vi "lisa_functional_3.vi"   [LabVIEW 2019]
doc: "The classic \"Hello World\" example."
uses:
  <vilib>/Analysis/Matrix/Datatypes/ComplexMatrix.ctl
  <vilib>/Analysis/Matrix/NI_Matrix.lvlib
types:
  T1 = typedef "imagedata.ctl" = cluster{"image type":i32, "image depth":i32, "image":u8[], "mask":u8[], "colors":u32[], "Rectangle":cluster{"left":i16, "top":i16, "right":i16, "bottom":i16}}
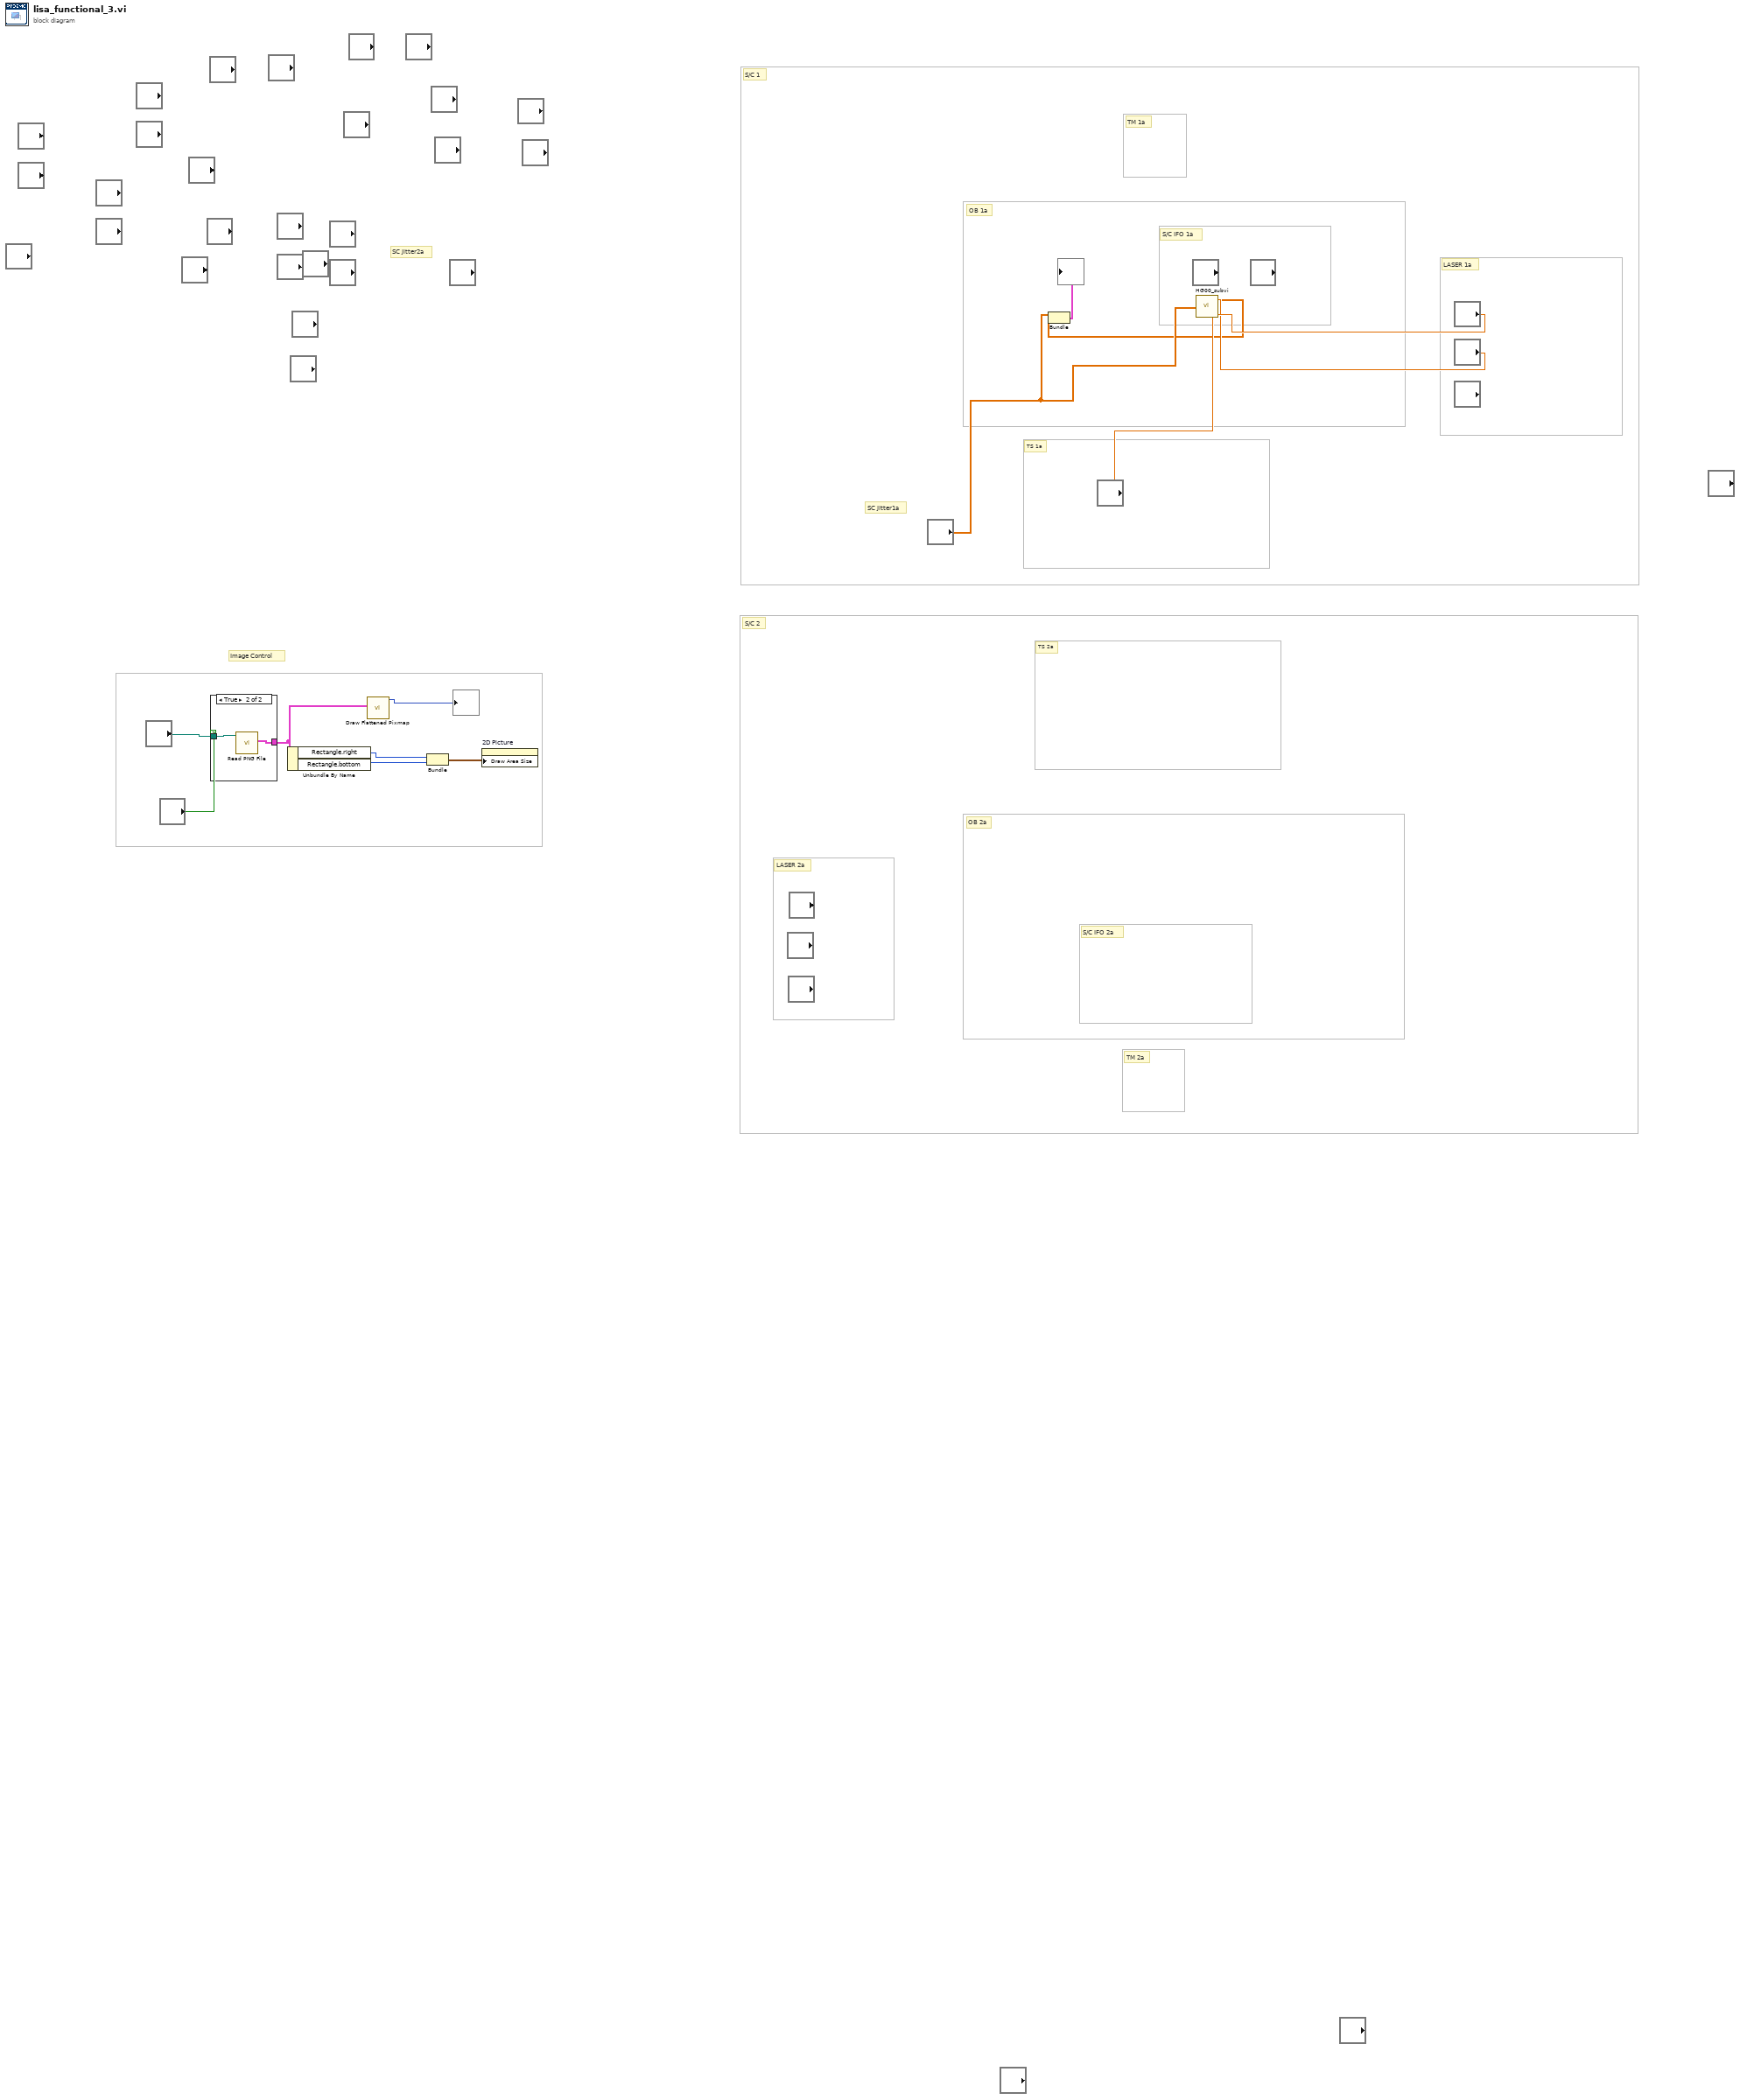
[diagram p0: block diagram]
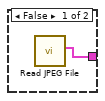
[diagram p2: hidden frame]
diagram:
  # "SC Jitter1a"
  # "SC Jitter2a"
  # "S/C IFO 2a"
  # "TM 2a"
  # "TS 2a"
  # "OB 2a"
  # "S/C 2"
  # "S/C IFO 1a"
  # "TM 1a"
  # "LASER 2a"
  # "Image Control"
  # "LASER 1a"
  # "TS 1a"
  # "OB 1a"
  # "S/C 1"
  n1 = case shown="True" "?" {
    tunnel: "?" -> [_ w16]
    tunnel: [w14 w15] -> w10
    frame False {
      n2 = call <vilib>:"Read JPEG File.vi"() -> ("image data"=w14:T1)  [unwired: 9 in, 2 out]
    }
    frame True {
      n3 = call <vilib>:"Read PNG File.vi"("path to PNG file"=w16) -> ("image data"=w15:T1)  [unwired: 8 in, 2 out]
    }
  }
  n4 = Unbundle By Name(w10) -> ("Rectangle.right"=w12:i16, "Rectangle.bottom"=w11:i16)
  n5 = call <vilib>:"Draw Flattened Pixmap.vi"("image data"=w10) -> ("new picture"=→"?":picture)  [unwired: 8 in]
  n6 = Bundle("right"=w12, "bottom"=w11) -> (w8:cluster{"right":i16, "bottom":i16})  [unwired: 1 in]
  n7 = property on="2D Picture" class="Pict"("Draw Area Size"=w8) -> ()  [unwired: 2 in, 2 out]
  n8 = call "HG00_subvi.vi"("Shift"="?", "Tilt"="?", "w"="?", "l"="?") -> ("return value 2"=w2:dbl[])  [unwired: 1 in]
  n9 = Bundle("a (t)"="?", "return value 2"=w2) -> (→"?":cluster{"a (t)":dbl[], "return value 2":dbl[]})  [unwired: 1 in]
